vi "Reports.Translate Folder of Results V1 ZIP to JSON File With Data Files.vi"() -> ()   [LabVIEW 2018]
panel:
  out "Total":i32
  out "Elapsed(s)":dbl format="%.2f"
  out "Numeric":i32
  out "error out":errorcluster
  in  "JSONOutDir":path
  in  "TempDir":path=path "C:/MTE/Translate/Temp"
  in  "Input Folder":path
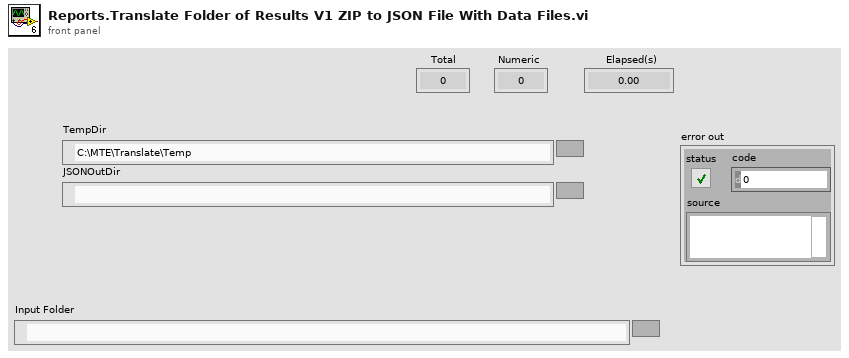
[diagram p1: front panel]
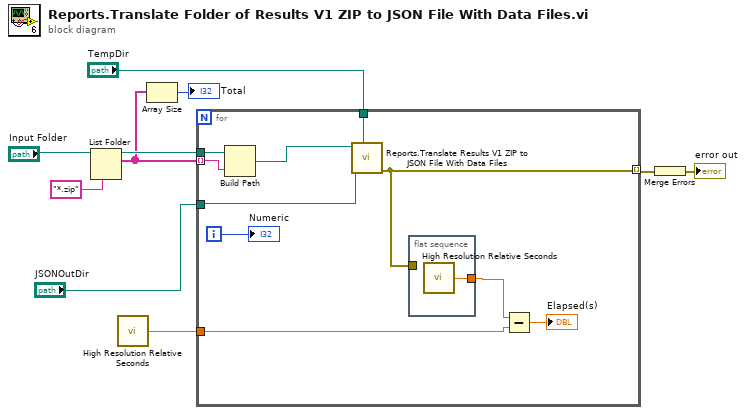
[diagram p0: block diagram]
diagram:
  n1 = List Folder(path="Input Folder", pattern="*.zip") -> (path out=w8:path, filenames=w1:string[])  [unwired: 2 in, 2 out]
  n2 = call <vilib>:"High Resolution Relative Seconds.vi"() -> ("relative seconds"=w3:dbl)
  n3 = Array Size(array=w1) -> (size(s)=→"Total":i32)
  n4 = for {
    tunnel: w8 -> [w20]
    tunnel: w1 -> [w19] mode=indexing
    tunnel: "TempDir" -> [w18]
    tunnel: "JSONOutDir" -> [w16]
    tunnel: [w14] -> w5 mode=indexing
    tunnel: w3 -> [w12]
    i -> [w15]
    n5 = Build Path(base path=w20, name or relative path=w19) -> (appended path=w17:path)
    n6 = call "Reports.Translate Results V1 ZIP to JSON File With Data Files.vi"("TempDir"=w18, "JSONOutDir"=w16, "ZipFileIn"=w17) -> ("error out"=w14:errorcluster)  [unwired: 8 in]
    n7 = flat-sequence {
      tunnel: w14 -> [_]
      tunnel: [w21] -> w13
      frame #0 {
        n8 = call <vilib>:"High Resolution Relative Seconds.vi"() -> ("relative seconds"=w21:dbl)
      }
    }
    n9 = Subtract(x=w13, y=w12) -> (x-y=→"Elapsed(s)":dbl)
    "Numeric" <- w15
  }
  n10 = Merge Errors(w5) -> (→"error out":errorcluster)
